vi "main.vi"() -> ()   [LabVIEW 2019]
uses:
  Controls/States.ctl
  Controls/Data.ctl
panel:
  out "Textout":string
  in  "Textin":string
  in  "Do Something":bool
  in  "Do Something Else":bool
  in  "Exit":bool
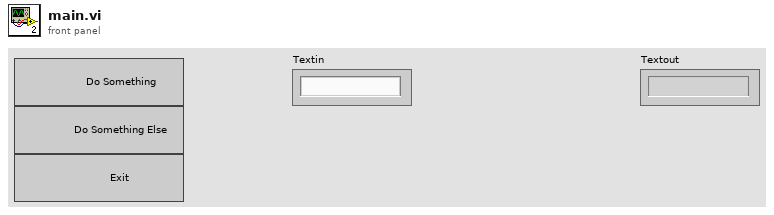
[diagram p1: front panel]
types:
  T1 = typedef "Data.ctl" = cluster{"Data":dbl[], "Info":string}
  T2 = typedef "States.ctl" = enum16{"Initialize", "Wait for Event", "Do Something", "Do Something Else", "Exit"}
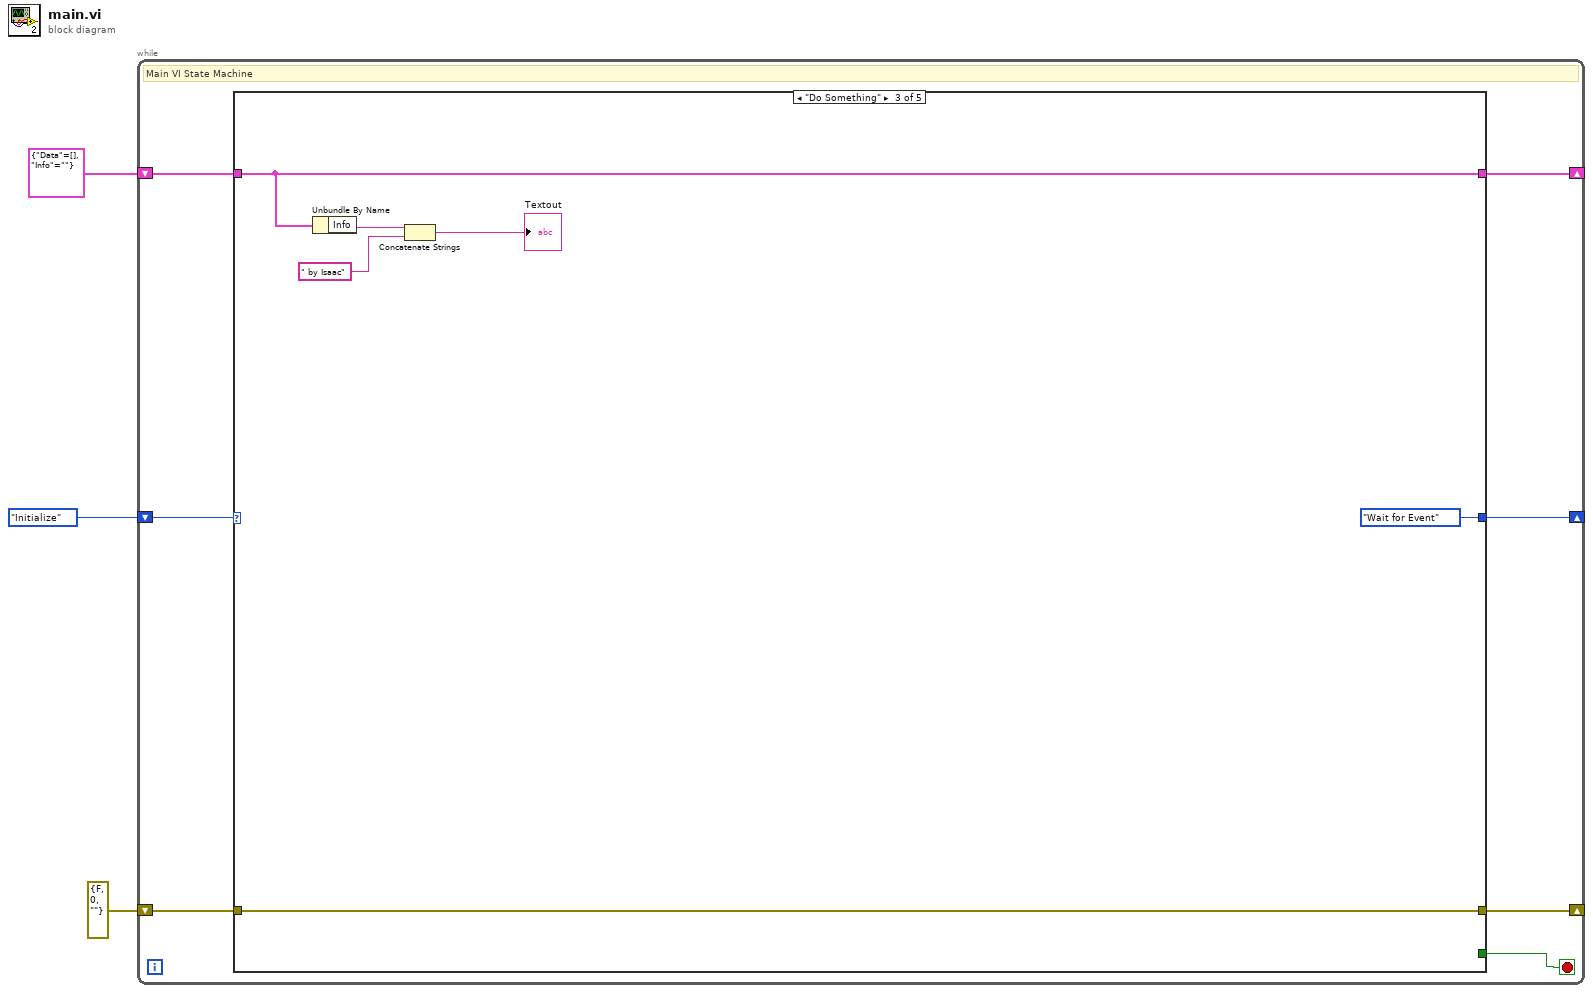
[diagram p0: block diagram]
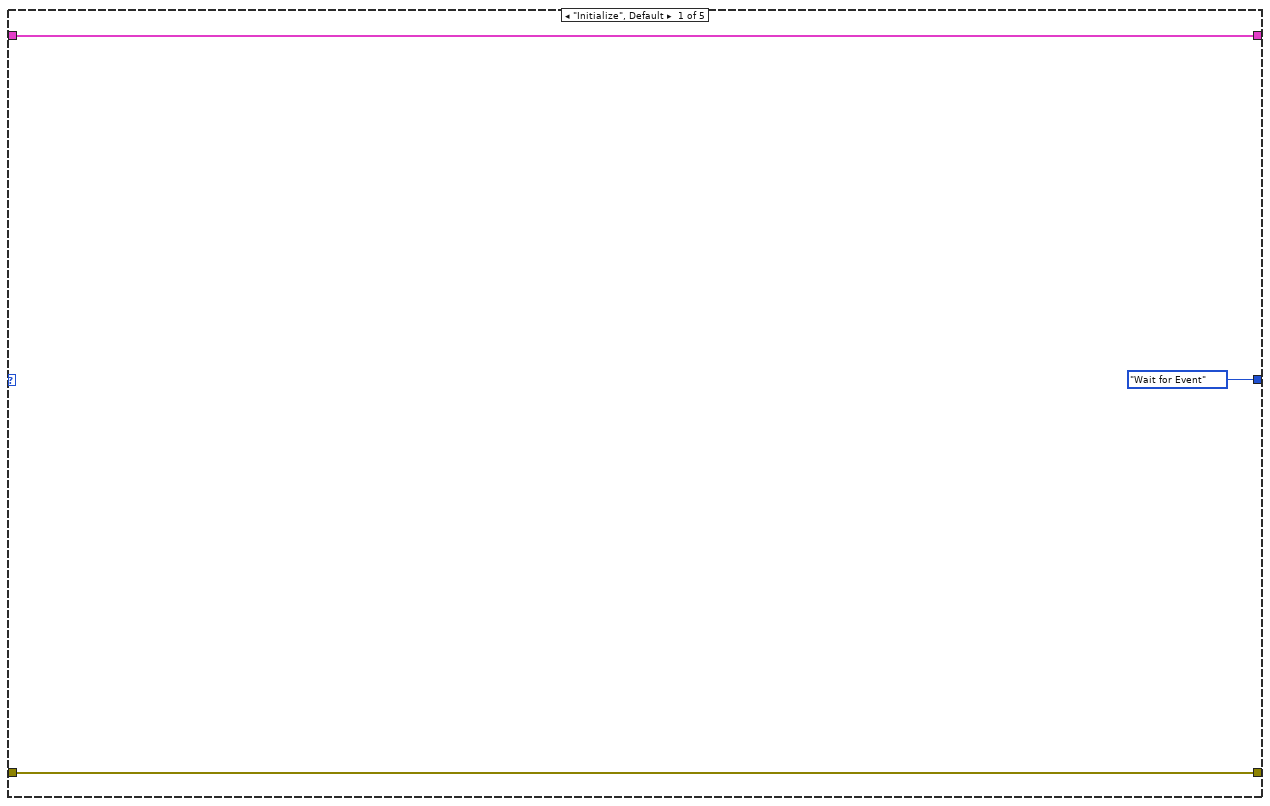
[diagram p2: hidden frame]
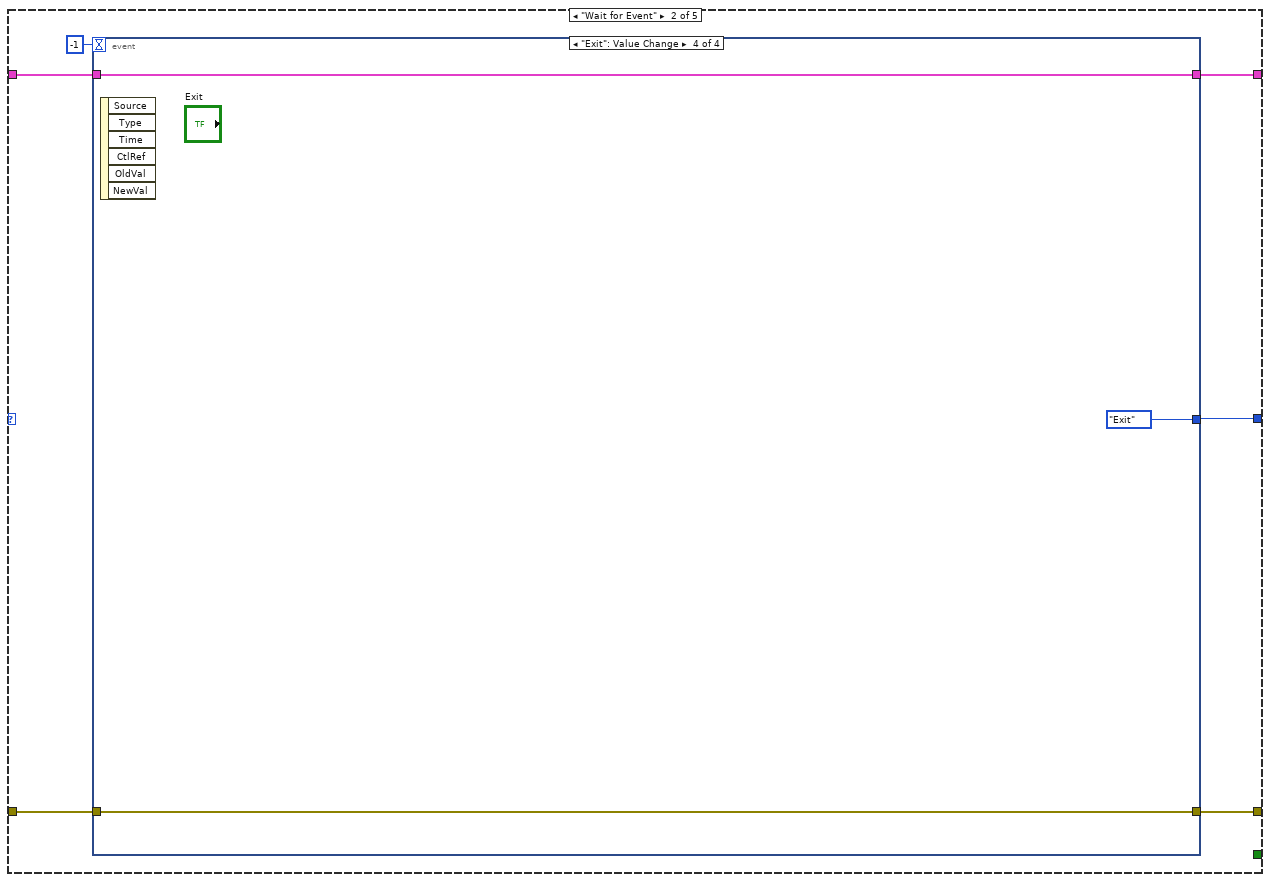
[diagram p3: hidden frame]
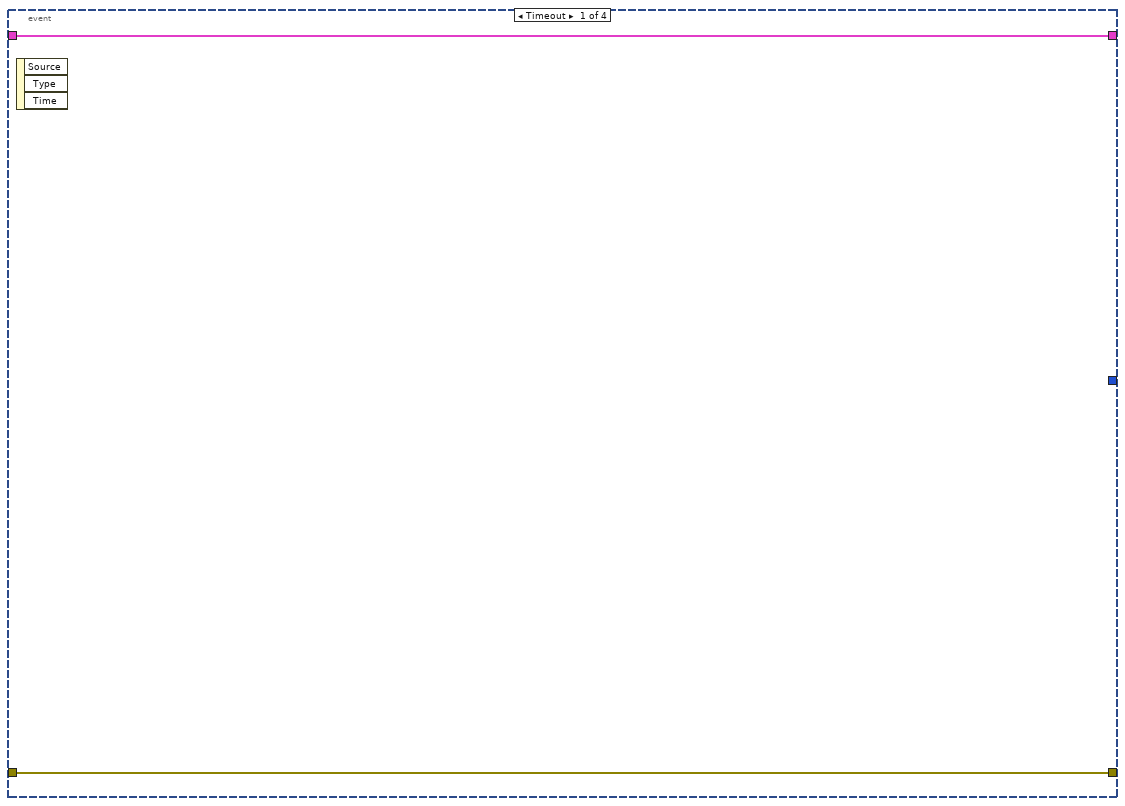
[diagram p4: hidden frame]
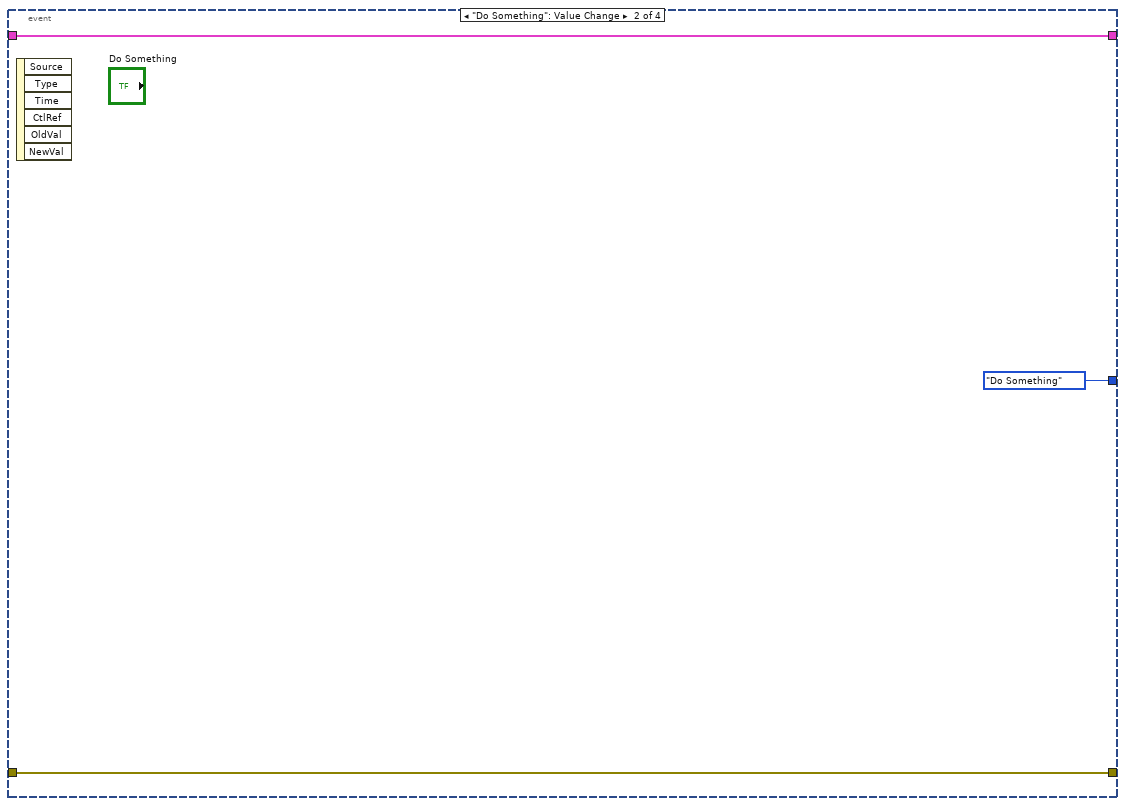
[diagram p5: hidden frame]
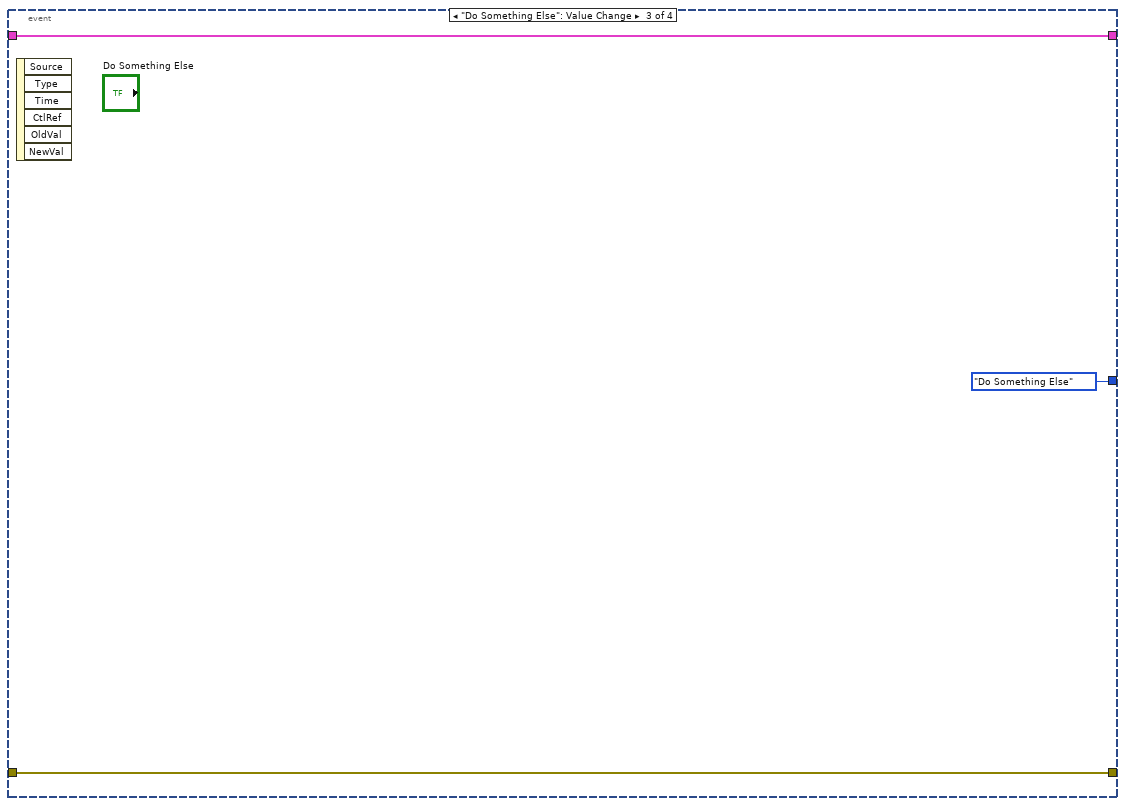
[diagram p6: hidden frame]
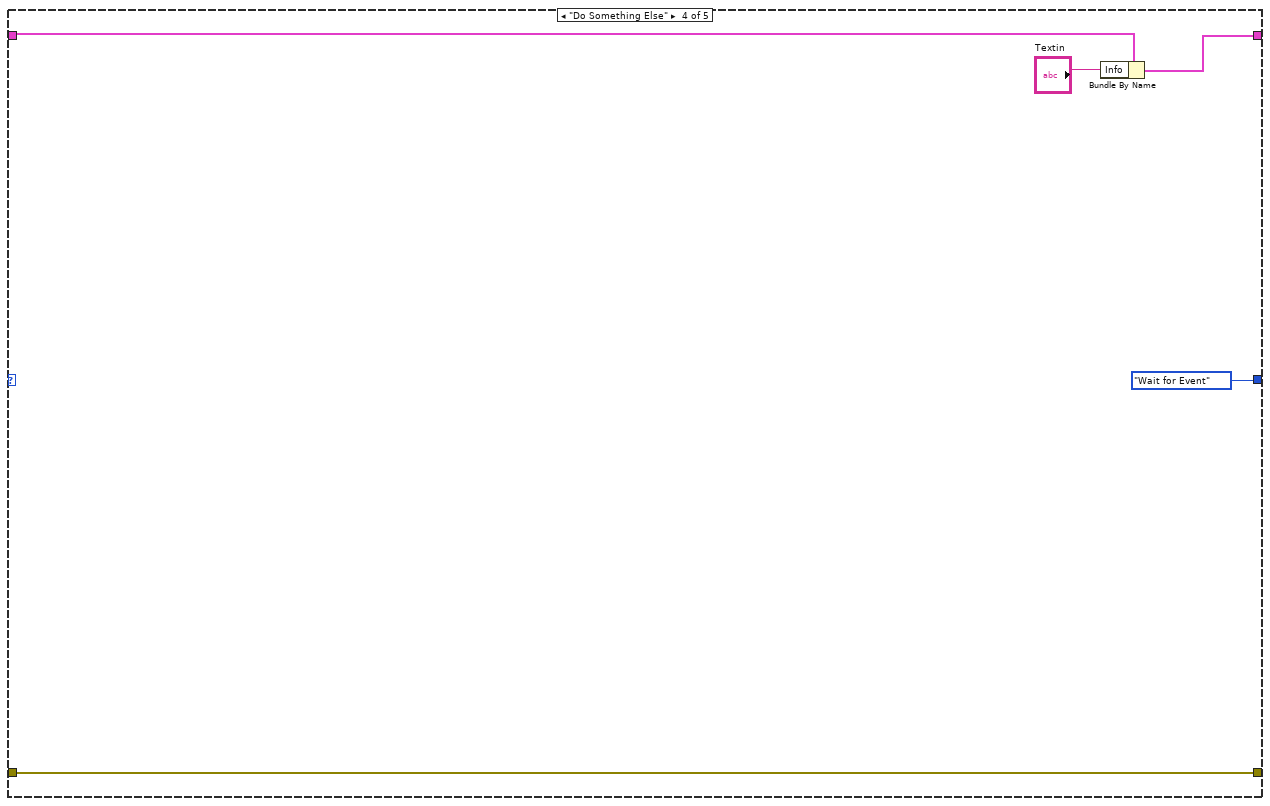
[diagram p7: hidden frame]
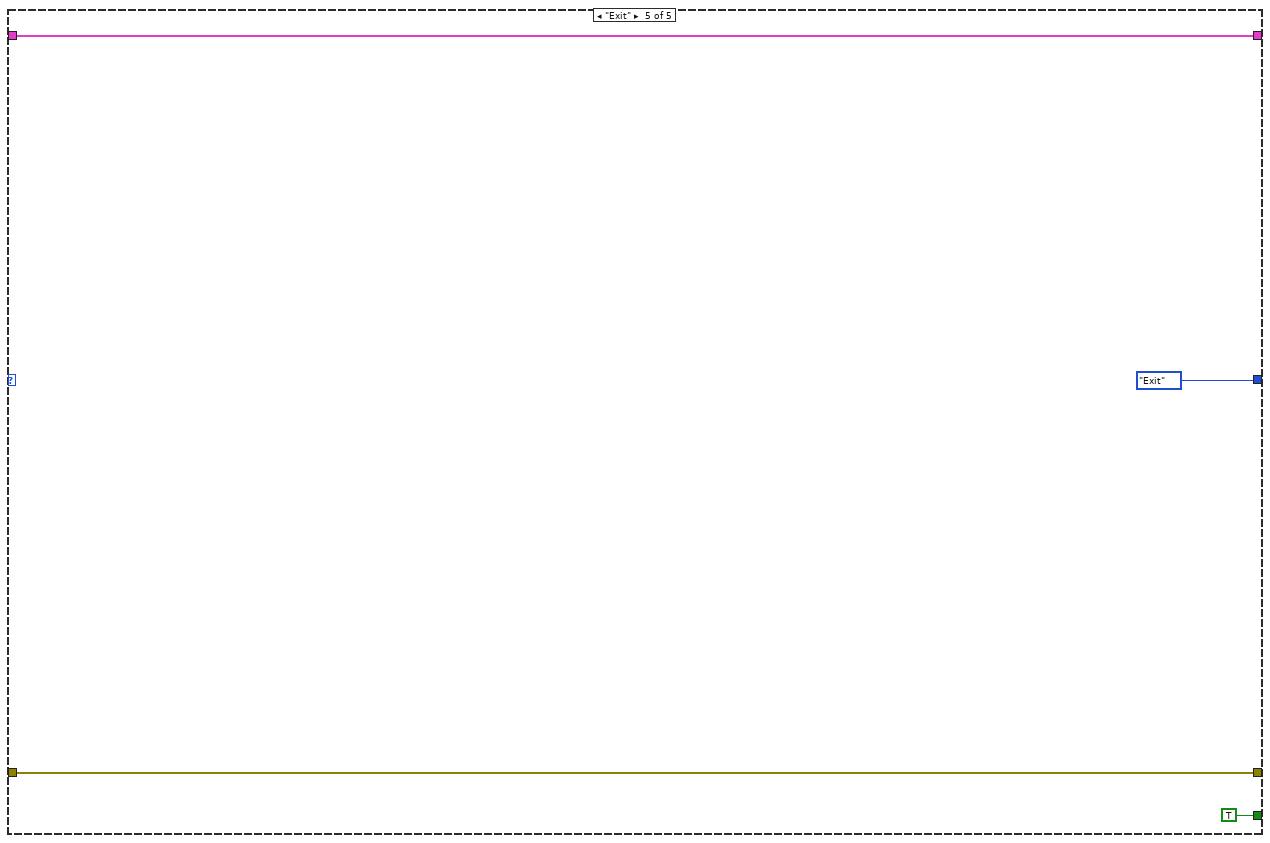
[diagram p8: hidden frame]
diagram:
  n1 = while {
    shift-right: [w9] -> _
    shift-left: States."Initialize" ("Enum") -> [w10]
    shift-right: [w6] -> _
    shift-left: T1 {"Data"=[], "Info"=""} ("Data") -> [w7]
    shift-right: [w4] -> _
    shift-left: errorcluster {"status"=FALSE, "code"=0, "source"=""} ("error constant") -> [w5]
    stop <- w8 stop-if-true
    # "Main VI State Machine"
    n2 = case shown="\"Do Something\"" w10 {
      tunnel: [States."Wait for Event" ("Enum") w19 States."Wait for Event" ("Enum") States."Wait for Event" ("Enum") States."Exit" ("Enum")] -> w9
      tunnel: [_ _ _ _ TRUE] -> w8
      tunnel: w7 -> [w12 w18 w34 w39 w43]
      tunnel: [w12 w17 w34 w37 w43] -> w6
      tunnel: w5 -> [w11 w15 w35 w40 w42]
      tunnel: [w11 w16 w35 w40 w42] -> w4
      frame "Initialize", Default {
      }
      frame "Wait for Event" {
        n3 = event shown="[3] \"Exit\": Value Change" {
          selector: _ -> [_ _ _ _]
          dyn-events: _ -> [_ _ _ _]
          timeout: -1 -> [_ _ _ _]
          tunnel: [_ States."Do Something" ("Enum") States."Do Something Else" ("Enum") States."Exit" ("Enum")] -> w19
          tunnel: w18 -> [w21 w23 w26 w29]
          tunnel: [w21 w23 w26 w29] -> w17
          tunnel: [w20 w22 w25 w28] -> w16
          tunnel: w15 -> [w20 w22 w25 w28]
          event Timeout {
            n4 = event-data() -> ()  [unwired: 1 in, 3 out]
          }
          event "Do Something": Value Change {
            n5 = event-data() -> ()  [unwired: 1 in, 6 out]
          }
          event "Do Something Else": Value Change {
            n6 = event-data() -> ()  [unwired: 1 in, 6 out]
          }
          event "Exit": Value Change {
            n7 = event-data() -> ()  [unwired: 1 in, 6 out]
          }
        }
      }
      frame "Do Something" {
        n8 = Unbundle By Name(w34) -> ("Info"=w33:string)
        n9 = Concatenate Strings "Concatenate Strings"(w33, " by Isaac" ("string")) -> (→"Textout":string)
      }
      frame "Do Something Else" {
        n10 = Bundle By Name(cluster=w39, "Info"="Textin") -> (w37:T1)
      }
      frame "Exit" {
      }
    }
  }
